vi "acq.Foldername.vi"() -> (1 "foldernme":string)   [LabVIEW 2020]
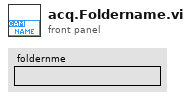
[diagram p1: front panel]
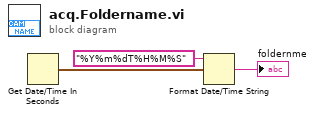
[diagram p0: block diagram]
diagram:
  n1 = Get Date/Time In Seconds() -> (seconds since 1Jan1904=w2:timestamp)
  n2 = Format Date/Time String(time format string (%c)="%Y%m%dT%H%M%S", seconds (now)=w2) -> (date/time string=→"foldernme":string)  [unwired: 1 in]
